vi "On Success.vi"(8 "error in (no error)":errorcluster, 9 "Session In":refnum<class "Session.lvclass">, 10 "User":refnum<class "User.lvclass">, 11 "SOL Auth in":refnum<class "SOL Auth.lvclass">) -> (0 "error out":errorcluster, 1 "Session":refnum<class "Session.lvclass">, 2 "Response":refnum<class "Response.lvclass">, 3 "SOL Auth out":refnum<class "SOL Auth.lvclass">)   [LabVIEW 2020, in "Summer of LabVIEW.lvlib" / "SOL Auth.lvclass"]
uses:
  SOL Auth.lvclass
  <vilib>/IlluminatedG/IG HTTP Utils/HTTP Utils/Response/Response.lvclass
  <vilib>/IlluminatedG/IG HTTP Server/HTTP Server/Session/Session.lvclass
  <vilib>/IlluminatedG/IG HTTP Server/HTTP Server/User/User.lvclass
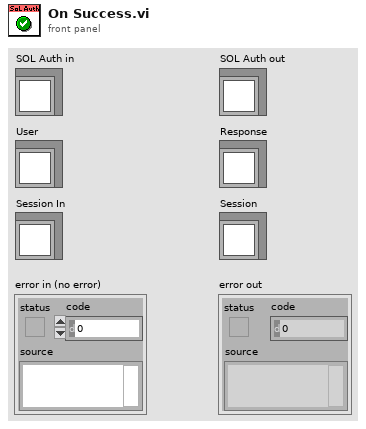
[diagram p1: front panel]
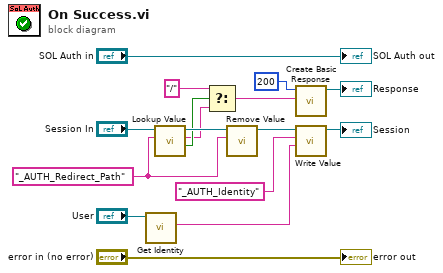
[diagram p0: block diagram]
diagram:
  w8 = "_AUTH_Redirect_Path" ("Name")
  n1 = call-dynamic "Get Identity.vi"("User in"="User") -> ("Identity"=w11:string)  [unwired: 8 in, 2 out]
  n2 = call <vilib>:"Lookup Value.vi"("Name"=w8, "Session in"="Session In") -> ("Not Found?"=w5:bool, "Value"=w4:string, "Session out"=w14:refnum<class "Session.lvclass">)  [unwired: 6 in, 1 out]
  n3 = Select(t="/", s=w5, f=w4) -> (s? t:f=w3:string)
  n4 = call <vilib>:"Remove Value.vi"("Name"=w8, "Session in"=w14) -> ("Session out"=w13:refnum<class "Session.lvclass">)  [unwired: 6 in, 3 out]
  n5 = call <vilib>:"Create Basic Response.vi"("Payload"=w3, "Status Code"=u16 200) -> ("Response out"=→"Response":refnum<class "Response.lvclass">)  [unwired: 8 in, 1 out]
  n6 = call <vilib>:"Write Value.vi"("Value"=w11, "Name"="_AUTH_Identity", "Session in"=w13) -> ("Session out"=→"Session":refnum<class "Session.lvclass">)  [unwired: 6 in, 2 out]
  "error out" <- "error in (no error)"
  "SOL Auth out" <- "SOL Auth in"
